vi "SEPW Specific Enthalpy of Pure Water (J to Kg).vi"(1 "Temp Pure Wate":dbl[unit]) -> (0 "SEPW":dbl[unit])   [LabVIEW 2018]
panel:
  out "Temprature of Pure Water \nKelvin Degree":dbl[unit](slide) scale=273.0..373.0
  out "Tk":dbl[unit]
  out "Temprature of Pure Water\nCentigrade Degree":dbl[unit](slide) scale=0.0..100.0
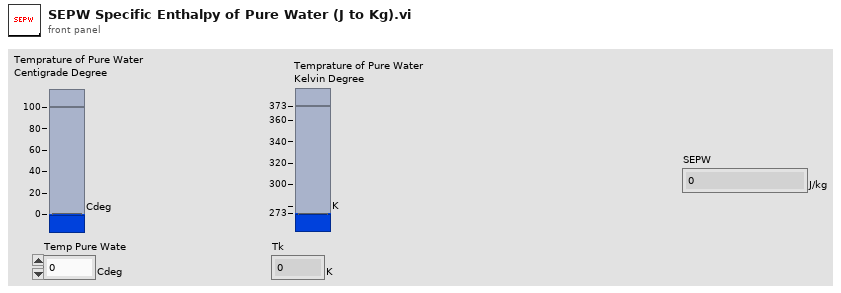
[diagram p1: front panel]
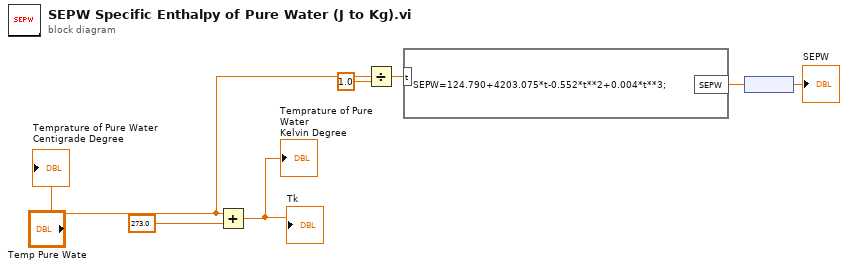
[diagram p0: block diagram]
diagram:
  n1 = Add(x="Temp Pure Wate", y=dbl[unit] 273.0) -> (x+y=→"Tk" →"Temprature of Pure Water \nKelvin Degree":dbl[unit])
  n2 = Divide(x="Temp Pure Wate", y=dbl[unit] 1.0) -> (x/y=w7:dbl)
  n3 = formula code="SEPW=124.790+4203.075*t-0.552*t**2+0.004*t**3;"("t"=w7) -> ("SEPW"=w5:dbl)
  n4 = node(w5) -> (→"SEPW":dbl[unit])
  "Temprature of Pure Water\nCentigrade Degree" <- "Temp Pure Wate"
